vi "Suma y tiempo de proceso.vi"() -> ()   [LabVIEW 2020]
panel:
  in  "stop":bool
  out "Numeric 4":dbl
  out "Numeric 3":dbl
  in  "Numeric 2":dbl
  in  "Numeric":dbl
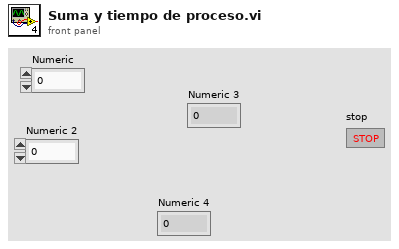
[diagram p1: front panel]
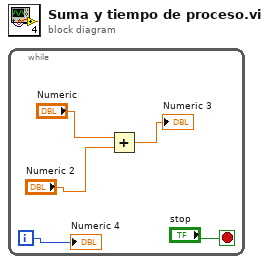
[diagram p0: block diagram]
diagram:
  n1 = while {
    i -> [w3]
    stop <- "stop" stop-if-true
    n2 = Add(x="Numeric", y="Numeric 2") -> (x+y=→"Numeric 3":dbl)
    "Numeric 4" <- w3
  }
